vi "ReadUntil.vi"(8 "error in (no error)":errorcluster, 9 "EOL":string, 10 "Console in":string, 11 "Python":T1) -> (0 "error out":errorcluster, 1 "timed out?":bool, 2 "Console out":string)   [LabVIEW 2021]
uses:
  PythonCtrl.ctl
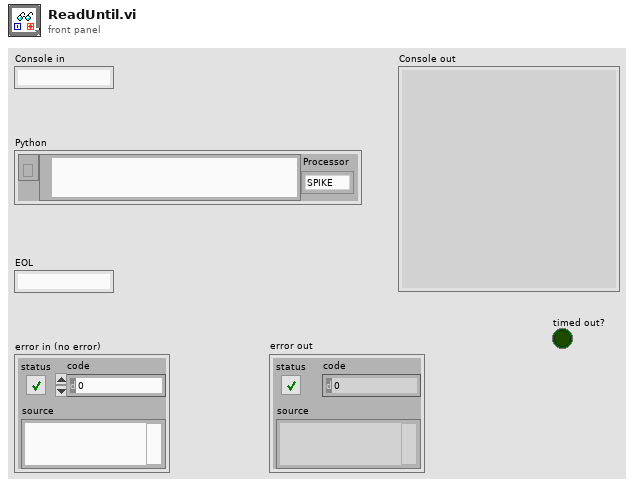
[diagram p1: front panel]
types:
  T1 = typedef "PythonCtrl.ctl" = cluster{"session":refnum<k35>, "PyPath":path, "Processor":enum16{"SPIKE", "Pi", "Pi_ssh"}}
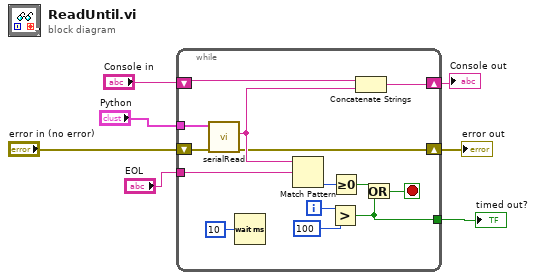
[diagram p0: block diagram]
diagram:
  n1 = while {
    tunnel: "Python" -> [w20]
    shift-right: [w17] -> w5
    shift-left: "Console in" -> [w18]
    tunnel: "EOL" -> [w10]
    shift-right: [w9] -> w2
    shift-left: "error in (no error)" -> [w21]
    tunnel: [w8] -> w1
    i -> [w14]
    stop <- w11 stop-if-true
    n2 = call "serialRead.vi"("error in (no error)"=w21, "Python"=w20) -> ("error out"=w9:errorcluster, "Reply"=w16:string)  [unwired: 7 in, 1 out]
    n3 = Wait (ms)(milliseconds to wait=u32 10) -> ()  [unwired: 1 out]
    n4 = Match Pattern(string=w16, regular expression=w10) -> (offset past match=w19:i32)  [unwired: 1 in, 3 out]
    n5 = Greater?(x=w14, y=u32 100 ("milliseconds to wait")) -> (0:w8:bool)
    n6 = Greater Or Equal To 0?(x=w19) -> (x >= 0?=w12:bool)
    n7 = Concatenate Strings(w18, w16) -> (w17:string)
    n8 = Or(x=w12, y=w8) -> (x .or. y?=w11:bool)
  }
  "Console out" <- w5
  "error out" <- w2
  "timed out?" <- w1
